vi "Eliminated.vi"(6 "Column":i32, 8 "Row":i32, 9 "Killer":i32, 10 "Team":i32, 11 "Experience in":refnum<class "Experience.lvclass">) -> (3 "Experience out":refnum<class "Experience.lvclass">)   [LabVIEW 2015, in "Experience.lvclass"]
uses:
  Experience.lvclass
  Square/Square.lvclass
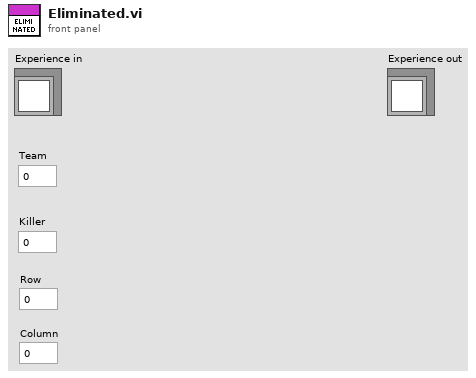
[diagram p1: front panel]
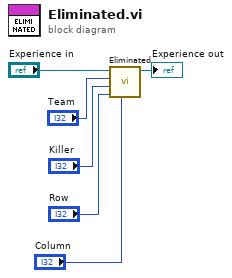
[diagram p0: block diagram]
diagram:
  n1 = call-parent "Eliminated.vi"("Column"="Column", "Row"="Row", "Killer"="Killer", "Team"="Team", "Square in"="Experience in") -> ("Square out"=→"Experience out":refnum<class "Experience.lvclass">)  [unwired: 6 in]
